vi "Dynamic Reset.vi"(0 "instrument handle":refnum<k15>, 2 "index":i32, 9 "RESET outfile":path=path "C:/Temp/RESET_out.tmp", 11 "error in (no error)":errorcluster, 12 "target resistance (ohm)":dbl=100000.0 format="%#_6p", 13 "Reset all others?":bool) -> (1 "SL voltage (V)":dbl, 3 "WL voltage (V)":dbl, 4 "instrument handle out":refnum<k15>, 6 "final resistance (ohm)":dbl format="%#_6p", 10 "final current (A)":dbl, 14 "reset?":bool, 15 "error out":errorcluster)   [LabVIEW 2018]
uses:
  Globals.vi
  <instrlib>/niDigital/niDigital.llb/niDigital Burst Pattern (Burst Only).vi
  <vilib>/Utility/file.llb/Write Delimited Spreadsheet (DBL).vi
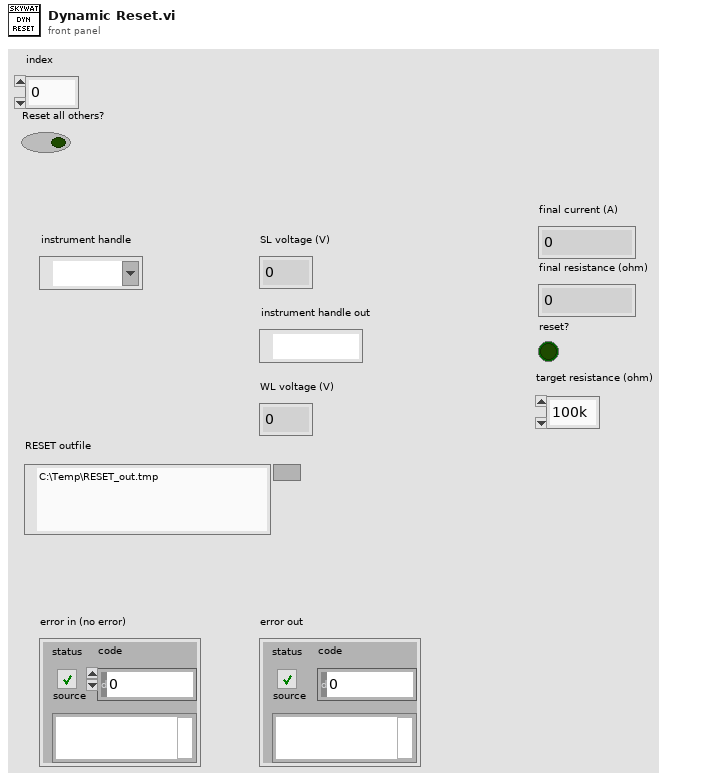
[diagram p1: front panel]
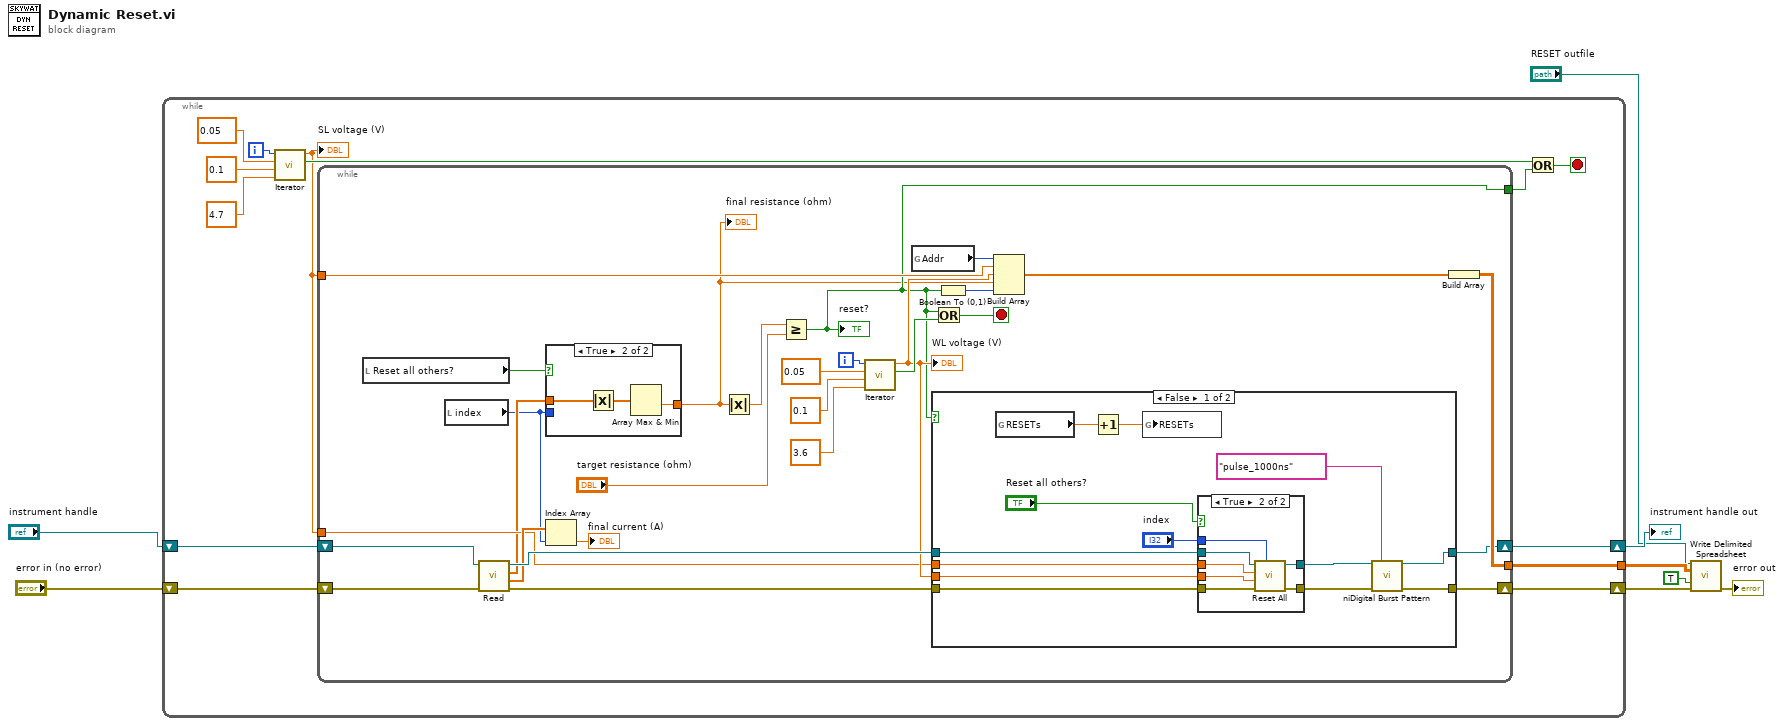
[diagram p0: block diagram]
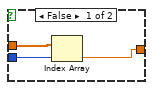
[diagram p2: hidden frame]
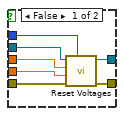
[diagram p3: hidden frame]
diagram:
  n1 = while {
    shift-right: [w17] -> w8
    shift-left: "instrument handle" -> [w15]
    shift-right: [w9] -> w3
    shift-left: "error in (no error)" -> [w14]
    tunnel: [w10] -> w5
    i -> [w18]
    stop <- w19 stop-if-true
    n2 = call "Iterator.vi"("Final Value"=4.7 ("y"), "Initial Value"=0.1 ("y"), "Step"=0.05 ("x"), "i"=w18) -> ("End Loop"=w16:bool, "Current Value"=w11:dbl)  [unwired: 6 in]
    "SL voltage (V)" <- w11
    n3 = while {
      shift-right: [w29] -> w17
      shift-left: w15 -> [w46]
      shift-right: [w30] -> w9
      shift-left: w14 -> [w26]
      tunnel: w11 -> [w36]
      tunnel: [w32] -> w12
      tunnel: w11 -> [w34]
      tunnel: [w31] -> w10
      i -> [w45]
      stop <- w49 stop-if-true
      n4 = local read "Reset all others?"() -> (w25:bool)
      n5 = local read "index"() -> (w23:i32)
      n6 = call "Read.vi"("error in (no error)"=w26, "instrument handle"=w46) -> ("error out"=w48:errorcluster, "currents (A)"=w40:dbl[], "resistances (ohm)"=w24:dbl[], "instrument handle out"=w47:refnum<k15>)  [unwired: 6 in]
      n7 = case shown="True" w25 {
        tunnel: w24 -> [w52 w54]
        tunnel: w23 -> [w51 _]
        tunnel: [w50 w55] -> w22
        frame False {
          n8 = Index Array(array=w52, index=w51) -> (element=w50:dbl)
        }
        frame True {
          n9 = Absolute Value(x=w54) -> (abs(x)=w53:dbl[])
          n10 = Array Max & Min(array=w53) -> (min value=w55:dbl)  [unwired: 3 out]
        }
      }
      "final resistance (ohm)" <- w22
      n11 = Index Array(array=w40, index=w23) -> (element=→"final current (A)":dbl)
      n12 = Absolute Value(x=w22) -> (abs(x)=w28:dbl)
      n13 = Greater Or Equal?(x=w28, y="target resistance (ohm)") -> (x >= y?=w32:bool)
      "reset?" <- w32
      n14 = call "Iterator.vi"("Final Value"=3.6 ("y"), "Initial Value"=0.1 ("y"), "Step"=0.05 ("x"), "i"=w45) -> ("End Loop"=w41:bool, "Current Value"=w35:dbl)  [unwired: 6 in]
      "WL voltage (V)" <- w35
      n15 = global read "Globals.vi" "Addr"() -> (w27:i32)
      n16 = case shown="False" w32 {
        tunnel: [w66 w83] -> w30
        tunnel: [w67 w84] -> w29
        tunnel: w48 -> [w60 w83]
        tunnel: w47 -> [w61 w84]
        tunnel: w35 -> [w58 _]
        tunnel: w34 -> [w59 _]
        frame False {
          n17 = global read "Globals.vi" "RESETs"() -> (w65:dbl)
          n18 = Increment(x=w65) -> (x+1=w64:dbl)
          n19 = global write "Globals.vi" "RESETs"(w64) -> ()
          n20 = case shown="True" "Reset all others?" {
            tunnel: [w75 w81] -> w63
            tunnel: [w74 w82] -> w62
            tunnel: w61 -> [w73 w79]
            tunnel: w60 -> [w72 w76]
            tunnel: w59 -> [w71 w77]
            tunnel: w58 -> [w70 w78]
            tunnel: "index" -> [w69 w80]
            frame False {
              n21 = call "Reset Voltages.vi"("index"=w69, "error in (no error)"=w72, "WL Voltage (V)"=w70, "SL Voltage (V)"=w71, "IVI Refnum in"=w73) -> ("error out"=w74:errorcluster, "IVI Refnum out"=w75:refnum<k15>)  [unwired: 5 in]
            }
            frame True {
              n22 = call "Reset All.vi"("index"=w80, "error in (no error)"=w76, "WL Voltage (V)"=w78, "SL Voltage (V)"=w77, "IVI Refnum in"=w79) -> ("error out"=w82:errorcluster, "IVI Refnum out"=w81:refnum<k15>)  [unwired: 5 in]
            }
          }
          n23 = call-poly <instrlib>:"niDigital Burst Pattern.vi"("instrument handle"=w63, "start label"="pulse_1000ns", "error in"=w62) -> ("instrument handle out"=w67:refnum<k15>, "error out"=w66:errorcluster)  [unwired: 11 in]
        }
        frame True {
        }
      }
      n24 = Or(x=w32, y=w41) -> (x .or. y?=w49:bool)
      n25 = Boolean To (0,1)(Boolean=w32) -> (0, 1=w39:i16)
      n26 = Build Array(w27, w36, w35, w22, w39) -> (w38:dbl[])
      n27 = Build Array(w38) -> (w31:dbl[][])
    }
    n28 = Or(x=w16, y=w12) -> (x .or. y?=w19:bool)
  }
  "instrument handle out" <- w8
  n29 = call-poly <vilib>:"Write Delimited Spreadsheet.vi"("file path (dialog if empty)"="RESET outfile", "2D data"=w5, "append to file? (new file:F)"=TRUE, "error in (no error)"=w3) -> ("error out"=→"error out":errorcluster)  [unwired: 10 in, 1 out]
